vi "TrajConstraint_GetType.vi"(11 "Trajectory Constraint":variant) -> (1 "Type Fount":bool, 3 "Trajectory Constraint Type":T1)   [LabVIEW 2019, in "Trajectory_Library.lvlib"]
doc: "Determines the type of a passed trajectory constraint.\n\nParameters:\n -Constraint - Variant containing the constraint to determine the type.\n\nReturns:\n - TrajjectoryConstraintType -- Enum containing the constraint type\n - Type Found -- Returns TRUE if the variant is a valid constraint type."
uses:
  Trajectory_Library.lvlib
  <vilib>/Utility/Data Type/NI_Data Type.lvlib
  Enum/TRAJ_CONSTRAINT_TYPES_ENUM.ctl
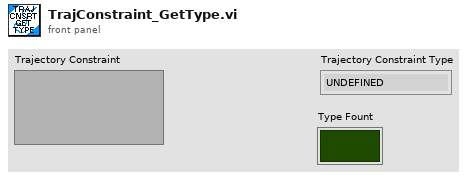
[diagram p1: front panel]
types:
  T1 = typedef "Trajectory_Library.lvlib/TRAJ_CONSTRAINT_TYPES_ENUM.ctl" = enum16{"UNDEFINED", "DIFF DRIVE KINEMATICS", "DIFF DRIVE VOLTAGE", "CENTRIPITAL ACCEL", "MECA DRIVE KINEMATICS", "SWERVE DRIVE KINEMATICS", "MAXIMUM VELOCITY", "ELLIPTICAL REGION", "RECTANGULAR REGION"}
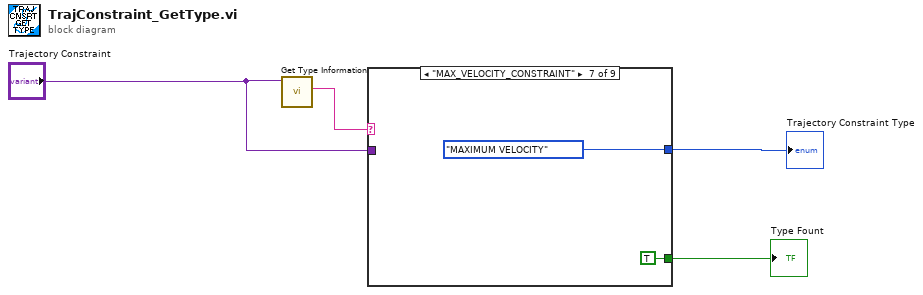
[diagram p0: block diagram]
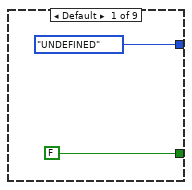
[diagram p2: hidden frame]
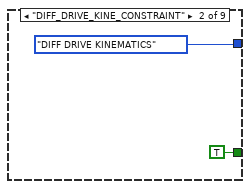
[diagram p3: hidden frame]
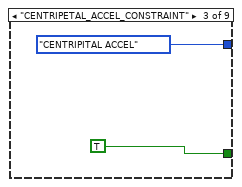
[diagram p4: hidden frame]
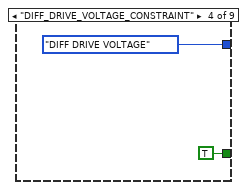
[diagram p5: hidden frame]
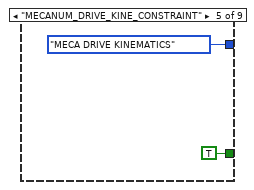
[diagram p6: hidden frame]
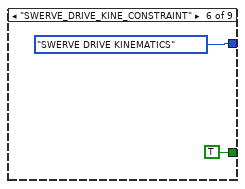
[diagram p7: hidden frame]
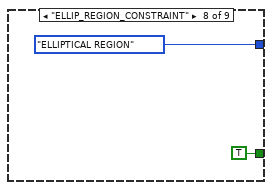
[diagram p8: hidden frame]
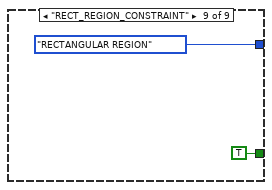
[diagram p9: hidden frame]
diagram:
  n1 = call <vilib>:"Get Type Information.vi"("variant"="Trajectory Constraint") -> ("name"=w3:string)  [unwired: 6 in, 4 out]
  n2 = case shown="\"MAX_VELOCITY_CONSTRAINT\"" w3 {
    tunnel: "Trajectory Constraint" -> [_ _ _ _ _ _ _ _ _]
    tunnel: [FALSE TRUE TRUE TRUE TRUE TRUE TRUE TRUE TRUE] -> w4
    tunnel: [TRAJ_CONSTRAINT_TYPES_ENUM."UNDEFINED" ("TRAJ_CONSTRAINT_TYPES") TRAJ_CONSTRAINT_TYPES_ENUM."DIFF DRIVE KINEMATICS" ("TRAJ_CONSTRAINT_TYPES") TRAJ_CONSTRAINT_TYPES_ENUM."CENTRIPITAL ACCEL" ("TRAJ_CONSTRAINT_TYPES") TRAJ_CONSTRAINT_TYPES_ENUM."DIFF DRIVE VOLTAGE" ("TRAJ_CONSTRAINT_TYPES") TRAJ_CONSTRAINT_TYPES_ENUM."MECA DRIVE KINEMATICS" ("TRAJ_CONSTRAINT_TYPES") TRAJ_CONSTRAINT_TYPES_ENUM."SWERVE DRIVE KINEMATICS" ("TRAJ_CONSTRAINT_TYPES") TRAJ_CONSTRAINT_TYPES_ENUM."MAXIMUM VELOCITY" ("TRAJ_CONSTRAINT_TYPES") TRAJ_CONSTRAINT_TYPES_ENUM."ELLIPTICAL REGION" ("TRAJ_CONSTRAINT_TYPES") TRAJ_CONSTRAINT_TYPES_ENUM."RECTANGULAR REGION" ("TRAJ_CONSTRAINT_TYPES")] -> w1
    frame Default {
    }
    frame "DIFF_DRIVE_KINE_CONSTRAINT" {
    }
    frame "CENTRIPETAL_ACCEL_CONSTRAINT" {
    }
    frame "DIFF_DRIVE_VOLTAGE_CONSTRAINT" {
    }
    frame "MECANUM_DRIVE_KINE_CONSTRAINT" {
    }
    frame "SWERVE_DRIVE_KINE_CONSTRAINT" {
    }
    frame "MAX_VELOCITY_CONSTRAINT" {
    }
    frame "ELLIP_REGION_CONSTRAINT" {
    }
    frame "RECT_REGION_CONSTRAINT" {
    }
  }
  "Trajectory Constraint Type" <- w1
  "Type Fount" <- w4
